vi "errstr.vi"(8 "error in (no error)":errorcluster, 11 "para0":i32) -> (0 "error out":errorcluster, 3 "function return":string)   [LabVIEW 2020, in "sqlite3.lvlib"]
uses:
  sqlite3.lvlib
  bin/sqlite3_64.dll
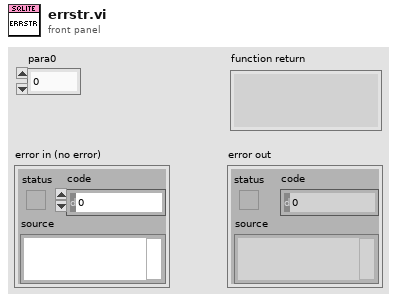
[diagram p1: front panel]
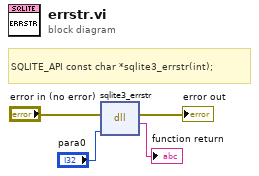
[diagram p0: block diagram]
diagram:
  # "SQLITE_API const char *sqlite3_errstr(int);"
  n1 = dll-call lib="D:/Project/Labview-Projects/database-configuration/externals/sqlite3/Source/bin/sqlite3_*.*" fn="sqlite3_errstr"(error in="error in (no error)", "para0"="para0") -> (error out=→"error out":errorcluster, →"function return":string)  [unwired: 3 in, 1 out]
